vi "DAQmx Create Channel (AI-Temperature-Thermistor-Vex).vi"(0 "task in":refnum<k21>, 1 "maximum value":dbl=100.0 format="%0.2f", 2 "minimum value":dbl format="%0.2f", 3 "resistance configuration":i32(ring)=4 items=["2-Wire"=2, "3-Wire"=3, "4-Wire"=4], 5 "physical channels":tag, 7 "name to assign":string, 9 "units":i32(ring)=10143 items=["Deg C"=10143, "Deg F"=10144, "Kelvins"=10325, "Deg R"=10145, "From Custom Scale"=10065], 10 "voltage excitation value":dbl=2.5 format="%0.5f", 11 "error in":errorcluster, 12 "thermistor characteristics":cluster{"A":dbl, "B":dbl, "C":dbl}={"A"=0.001295361, "B"=0.0002343159, "C"=1.018703e-07} {"C" format="%^0.7e"; "B" format="%^0.7e"; "A" format="%^0.7e"}, 13 "voltage excitation source":i32(ring)=10167 items=["Internal"=10200, "External"=10167, "None"=10230], 14 "r1":dbl=5000.0 format="%0.2f") -> (4 "task out":refnum<k21>, 15 "error out":errorcluster)   [LabVIEW 2020]
doc: "Creates channel(s) that use a thermistor to measure temperature. Use this instance when the thermistor requires voltage excitation."
uses:
  nilvaiu.dll
panel:
  # "input limits"
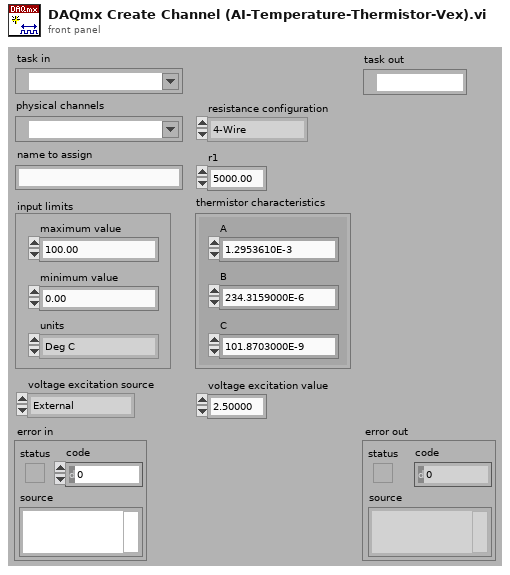
[diagram p1: front panel]
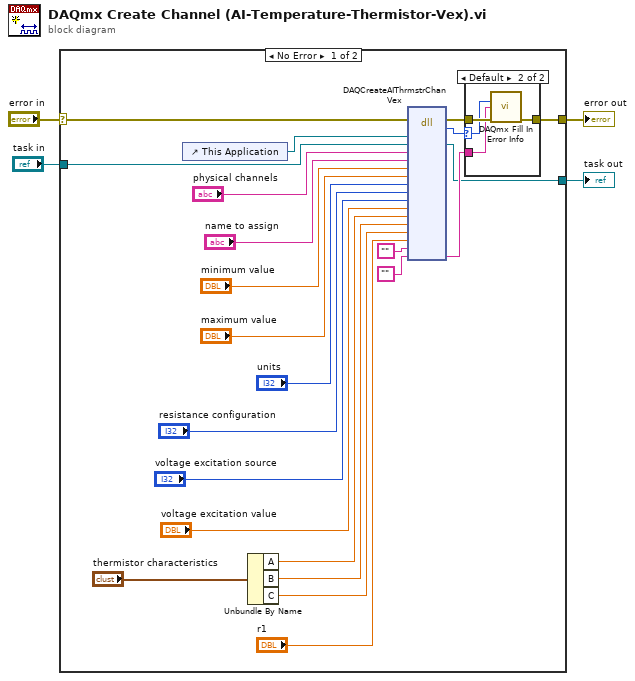
[diagram p0: block diagram]
diagram:
  n1 = case shown="No Error" "error in" {
    selector: "error in" -> [w8 w33]
    tunnel: "task in" -> [w10 w34]
    tunnel: [w9 w34] -> w3
    tunnel: [w7 w33] -> w1
    frame No Error {
      n2 = control-ref of="This Application"() -> (w11:refnum<vi>)
      n3 = Unbundle By Name("thermistor characteristics") -> ("A"=w17:dbl, "B"=w16:dbl, "C"=w15:dbl)
      n4 = dll-call lib="nilvaiu.*" fn="DAQCreateAIThrmstrChanVex"(error in=w8, "lvAppRef"=w11, "refObjPtr"=w10, "physicalChannelName"="physical channels", "channelNameIn"="name to assign", "minVal"="minimum value", "maxVal"="maximum value", "units"="units", "resistanceConfig"="resistance configuration", "voltageExcitSource"="voltage excitation source", "voltageExcitVal"="voltage excitation value", "a"=w17, "b"=w16, "c"=w15, "r1"="r1", "channelNamesOut"="", "extended error info"="") -> (error out=w27:errorcluster, "return type"=w25:i32, "refObjPtr"=w9:refnum<k21>, "extended error info"=w26:string)  [unwired: 16 in, 1 out]
      n5 = case shown="Default" w25 {
        selector: w25 -> [_ w30]
        tunnel: w27 -> [w28 w32]
        tunnel: [w28 w31] -> w7
        tunnel: w26 -> [_ w29]
        frame 0 {
        }
        frame Default {
          n6 = call "DAQmx Fill In Error Info.vi"("status code"=w30, "extended error info"=w29, "error in"=w32) -> ("error out"=w31:errorcluster)  [unwired: 1 in, 11 out]
        }
      }
    }
    frame Error {
    }
  }
  "task out" <- w3
  "error out" <- w1
